vi "DefendGoalTacticCheckStateChange.vi"(8 "error in (no error)":errorcluster, 10 "Game":refnum<class "Game.lvclass">, 11 "DefendGoalTactic in":refnum<class "DefendGoalTactic.lvclass">) -> (0 "error out":errorcluster, 2 "States":T1(ring), 3 "DefendGoalTactic out":refnum<class "DefendGoalTactic.lvclass">)   [LabVIEW 2023, in "DefendGoalTactic.lvclass"]
uses:
  DefendGoalTactic.lvclass
  Game_class/Game.lvclass
  Referee_class/command_interpreted.ctl
  Game_class/Game.lvclass/Game.ctl
  Referee_class/Referee.lvclass/Referee.ctl
  Events_class/Events.lvclass/Events.ctl
  Ball_class/Ball.lvclass/Ball.ctl
  Parameters_class/Parameters.lvclass/Parameters.ctl
  Team_class/Team.lvclass/Team.ctl
  Team_class/Read RobotRef.vi
  Referee_class/Read our_goalie_id.vi
  Game_class/Read Referee.vi
  Game_class/Read AllyRef.vi
  Game_class/Read Utilities.lvclass.vi
  Game_class/Read EnemyRef.vi
  Game_class/Read EventsRef.vi
  Game_class/Read BallRef.vi
  Game_class/Read Parameters.lvclass.vi
  Parameters_class/Read AttakingOurselves.vi
  Ball_class/Read v_x.vi
  Ball_class/Read v_y.vi
  Events_class/Read ball_inside_our_goalie_area.vi
  Referee_class/Read command_interpreted.vi
  Enemy_class/Enemy.lvclass
  Ally_class/Ally.lvclass
  Referee_class/Referee.lvclass
  Utilities_class/Utilities.lvclass
  Events_class/Events.lvclass
  Ball_class/Ball.lvclass
  Parameters_class/Parameters.lvclass
  Robot_class/Robot.lvclass
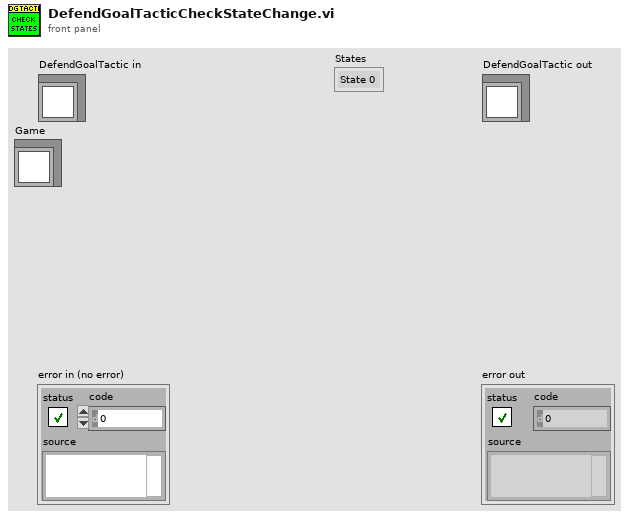
[diagram p1: front panel]
types:
  T1 = enum16{"State 0", "State 1", "State 2", "State 3", "Exit"}
  T2 = typedef "command_interpreted.ctl" = enum16{"Goal Ally", "Goal Enemy", "Ball Placement Enemy", "Ball Placement Ally", "Normal Half Time", "Extra Time  Break", "Extra Half Time", "None", "Post Game", "PKA Normal Start", "Prepare Kickoff Ally", "PKE Normal Start", "Prepare Kickoff Enemy", "Force Start", "Halt", "Timeout", "Prepare Penalty Ally", "Prepare Penalty Enemy", "PPA NormalStart", "PPE Normal Start", "Indirect Free Ally", "Direct Free Enemy", "Direct Free Ally", "Indirect Free Enemy", "Stop"}
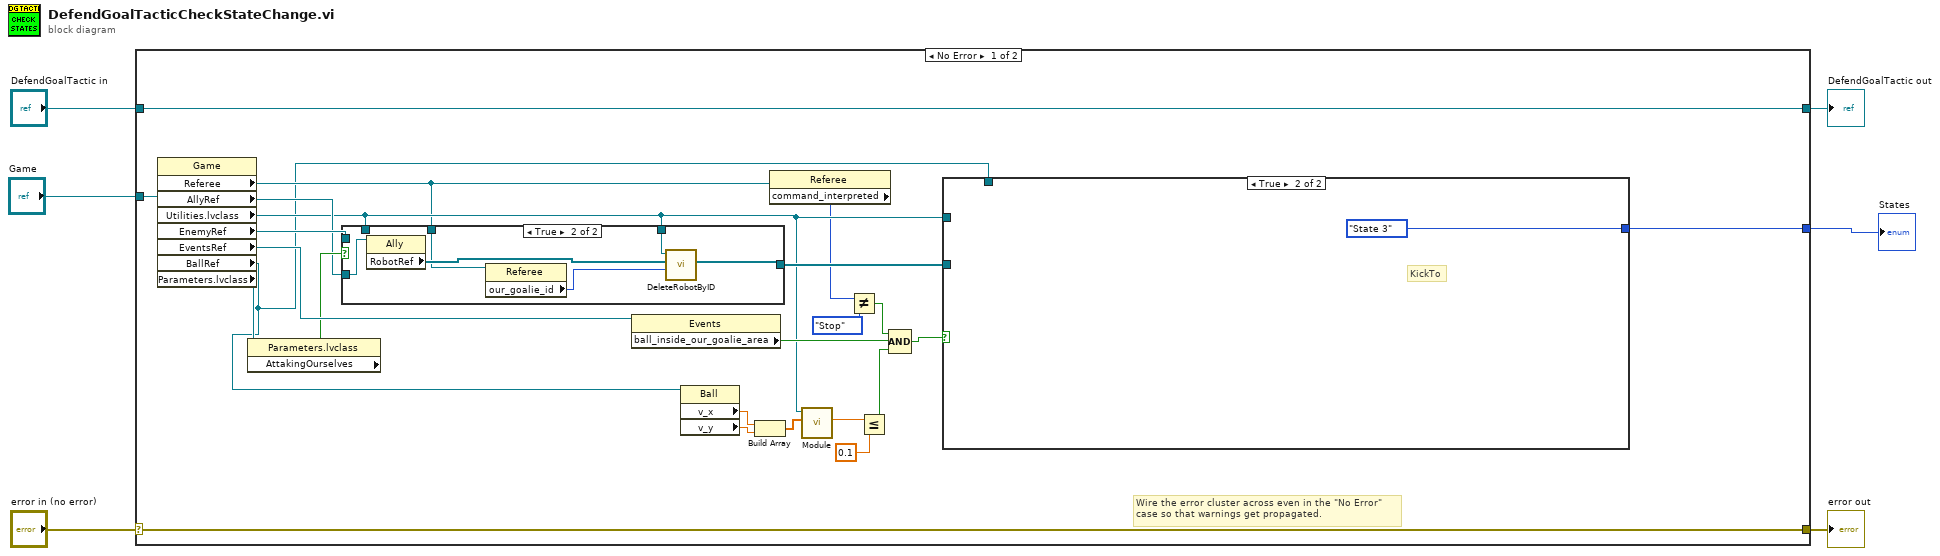
[diagram p0: block diagram]
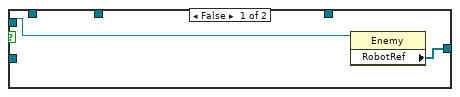
[diagram p2: hidden frame]
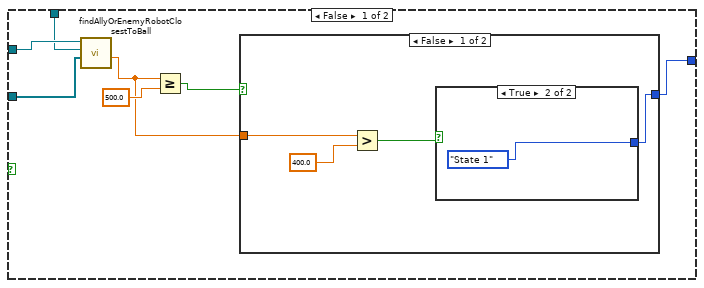
[diagram p3: hidden frame]
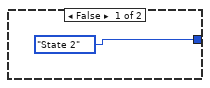
[diagram p4: hidden frame]
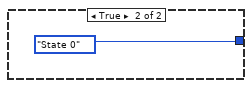
[diagram p5: hidden frame]
diagram:
  n1 = case shown="No Error" "error in (no error)" {
    selector: "error in (no error)" -> [w29 w55]
    tunnel: [w29 w55] -> w5
    tunnel: [w30 w54] -> w3
    tunnel: "DefendGoalTactic in" -> [w30 w54]
    tunnel: "Game" -> [w12 _]
    tunnel: [w27 _] -> w1
    frame No Error {
      # "Wire the error cluster across even in the \"No Error\"\ncase so that warnings get propagated."
      n2 = property class="Game"(reference=w12) -> ("Referee"=w11:refnum<class "Referee.lvclass">, "AllyRef"=w24:refnum<class "Ally.lvclass">, "Utilities.lvclass"=w13:refnum<class "Utilities.lvclass">, "EnemyRef"=w28:refnum<class "Enemy.lvclass">, "EventsRef"=w26:refnum<class "Events.lvclass">, "BallRef"=w7:refnum<class "Ball.lvclass">, "Parameters.lvclass"=w21:refnum<class "Parameters.lvclass">)  [unwired: 1 in, 2 out]
      n3 = property class="Parameters.lvclass"(reference=w21) -> ("AttakingOurselves"=w25:bool)  [unwired: 1 in, 2 out]
      n4 = case shown="True" w25 {
        tunnel: w28 -> [w32 _]
        tunnel: [w31 w33] -> w14
        tunnel: w24 -> [_ w38]
        tunnel: w13 -> [_ _]
        tunnel: w13 -> [_ w36]
        tunnel: w11 -> [_ w35]
        frame False {
          n5 = property class="Enemy"(reference=w32) -> ("RobotRef"=w31:refnum<class "Robot.lvclass">[])  [unwired: 1 in, 2 out]
        }
        frame True {
          n6 = property class="Ally"(reference=w38) -> ("RobotRef"=w37:refnum<class "Robot.lvclass">[])  [unwired: 1 in, 2 out]
          n7 = property class="Referee"(reference=w35) -> ("our_goalie_id"=w34:i32)  [unwired: 1 in, 2 out]
          n8 = call-dynamic "DeleteRobotByID.vi"("id"=w34, "RobotRef"=w37, "Utilities in"=w36) -> ("RobotRef out"=w33:refnum<class "Robot.lvclass">[])  [unwired: 6 in, 2 out]
        }
      }
      n9 = property class="Events"(reference=w26) -> ("ball_inside_our_goalie_area"=w23:bool)  [unwired: 1 in, 2 out]
      n10 = property class="Ball"(reference=w7) -> ("v_x"=w20:dbl, "v_y"=w19:dbl)  [unwired: 1 in, 2 out]
      n11 = Build Array(w20, w19) -> (w18:dbl[])
      n12 = property class="Referee"(reference=w11) -> ("command_interpreted"=w10:T2)  [unwired: 1 in, 2 out]
      n13 = call-dynamic "Module.vi"("2D vector"=w18, "Utilities in"=w13) -> ("Modulo"=w17:dbl)  [unwired: 7 in, 2 out]
      n14 = Not Equal?(x=w10, y=command_interpreted."Stop") -> (x != y?=w8:bool)
      n15 = Less Or Equal?(x=w17, y=0.1) -> (x <= y?=w15:bool)
      n16 = Compound Arithmetic op=AND(w8, w23, w15) -> (w22:bool)
      n17 = case shown="True" w22 {
        tunnel: [w45 T1."State 3" ("States")] -> w27
        tunnel: w14 -> [w41 _]
        tunnel: w13 -> [w40 _]
        tunnel: w7 -> [w39 _]
        frame False {
          n18 = call "findAllyOrEnemyRobotClosestToBall.vi"("Ally/Enemy Robots"=w41, "Ball"=w39, "Utilities in"=w40) -> ("Robot distance to ball"=w42:dbl)  [unwired: 5 in, 3 out]
          n19 = Greater Or Equal?(x=w42, y=500.0) -> (x >= y?=w43:bool)
          n20 = case shown="False" w43 {
            tunnel: [w46 T1."State 0" ("States")] -> w45
            tunnel: w42 -> [w49 _]
            frame False {
              n21 = Greater?(x=w49, y=400.0) -> (0:w47:bool)
              n22 = case shown="True" w47 {
                tunnel: [T1."State 2" ("States") T1."State 1" ("States")] -> w46
                frame False {
                }
                frame True {
                }
              }
            }
            frame True {
            }
          }
        }
        frame True {
          # "KickTo"
        }
      }
    }
    frame Error {
    }
  }
  "error out" <- w5
  "DefendGoalTactic out" <- w3
  "States" <- w1
